vi "GSE 350 Build Full Data String.vi"(8 "Error In":errorcluster, 9 "Latest Data":string, 10 "Previous Data":string, 11 "Full Data String Input":string) -> (0 "Error Out":errorcluster, 1 "Read Buffer (Out)":string, 2 "Full Data String":string, 3 "concatenated string":string)   [LabVIEW 2016]
panel:
  out "x != y? 3":bool
  out "x != y? 2":bool
  out "x != y?":bool
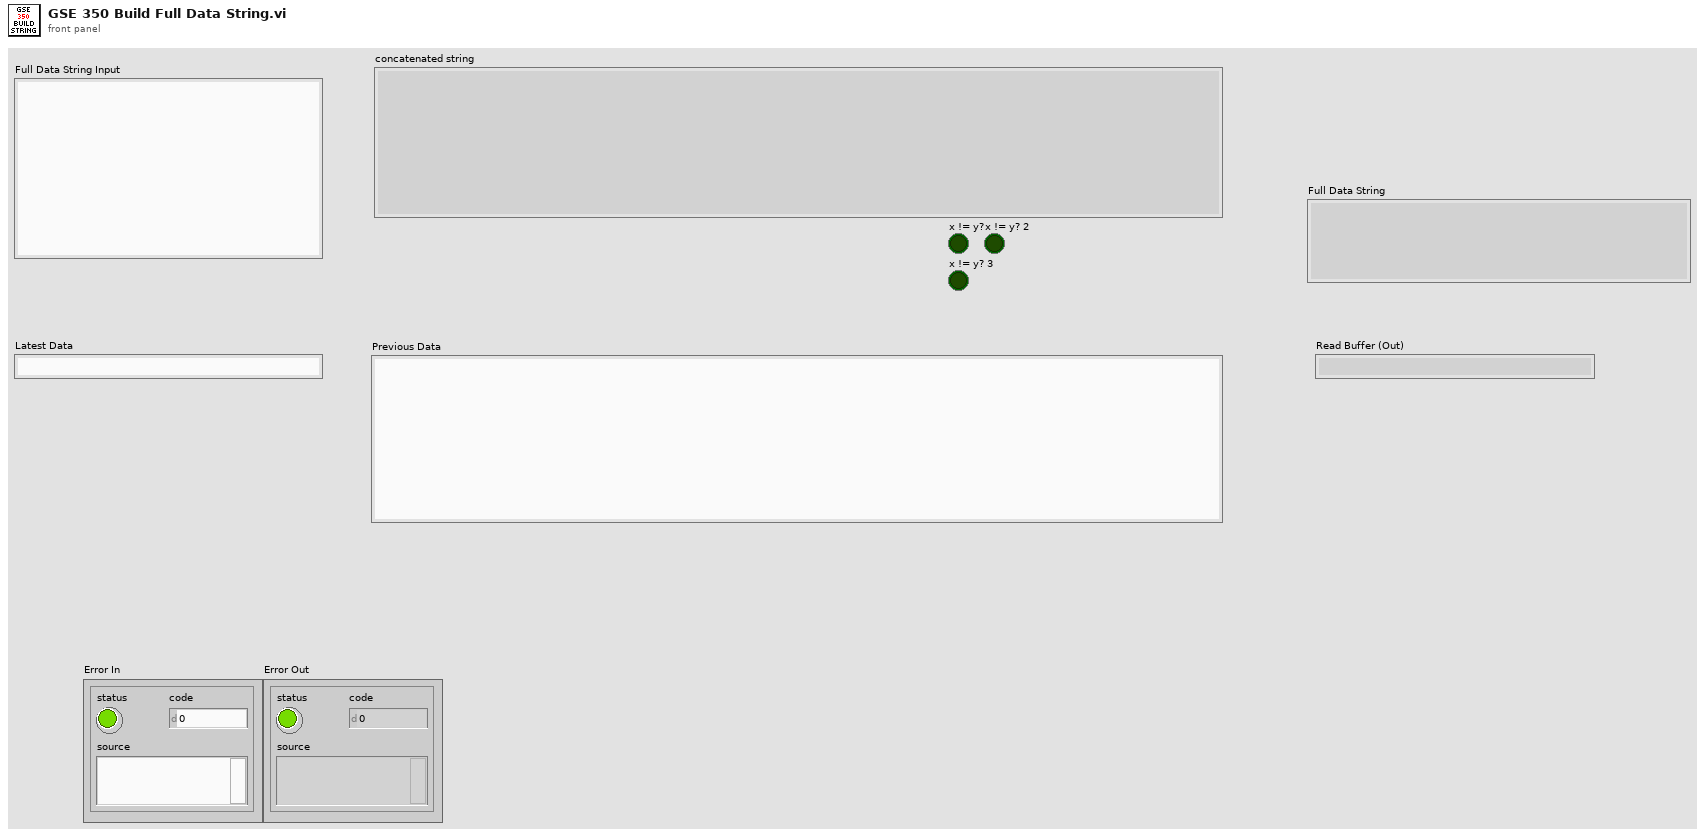
[diagram p1: front panel]
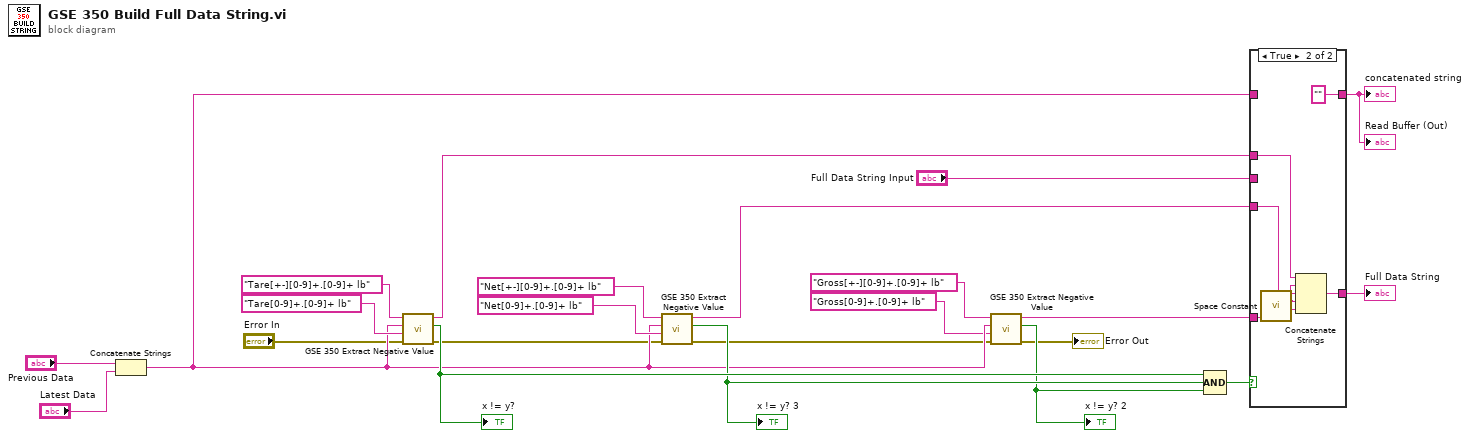
[diagram p0: block diagram]
diagram:
  n1 = Concatenate Strings("Previous Data", "Latest Data") -> (w9:string)
  n2 = call "GSE 350 Extract Negative Value.vi"("Error In"="Error In", "Regular Expression Search"="Tare[0-9]+.[0-9]+ lb" ("regular expression"), "Full String"=w9, "Expression With Negative Search"="Tare[+-][0-9]+.[0-9]+ lb" ("regular expression")) -> ("Error Out"=w4:errorcluster, "Found Match"=w14:bool, "Output Match"=w17:string)  [unwired: 4 in, 1 out]
  "x != y?" <- w14
  n3 = call "GSE 350 Extract Negative Value.vi"("Error In"=w4, "Regular Expression Search"="Net[0-9]+.[0-9]+ lb" ("regular expression"), "Full String"=w9, "Expression With Negative Search"="Net[+-][0-9]+.[0-9]+ lb" ("regular expression")) -> ("Error Out"=w3:errorcluster, "Found Match"=w10:bool, "Output Match"=w11:string)  [unwired: 4 in, 1 out]
  "x != y? 3" <- w10
  n4 = call "GSE 350 Extract Negative Value.vi"("Error In"=w3, "Regular Expression Search"="Gross[0-9]+.[0-9]+ lb" ("regular expression"), "Full String"=w9, "Expression With Negative Search"="Gross[+-][0-9]+.[0-9]+ lb" ("regular expression")) -> ("Error Out"=→"Error Out":errorcluster, "Found Match"=w5:bool, "Output Match"=w6:string)  [unwired: 4 in, 1 out]
  "x != y? 2" <- w5
  n5 = Compound Arithmetic op=AND(w14, w10, w5) -> (w18:bool)
  n6 = case shown="True" w18 {
    tunnel: w9 -> [w25 _]
    tunnel: [w25 ""] -> w16
    tunnel: [w24 w26] -> w23
    tunnel: "Full Data String Input" -> [w24 _]
    tunnel: w17 -> [_ w30]
    tunnel: w11 -> [_ w29]
    tunnel: w6 -> [_ w27]
    frame False {
    }
    frame True {
      n7 = call <vilib>:"Space Constant.vi"() -> ("String"=w28:string)
      n8 = Concatenate Strings(w30, w28, w29, w28, w27) -> (w26:string)
    }
  }
  "Full Data String" <- w23
  "Read Buffer (Out)" <- w16
  "concatenated string" <- w16
